vi "Unique.vi"(11 "Type in":refnum<class "Type.lvclass">) -> (2 "Unique":bool)   [LabVIEW 2020, in "Conditum.lvlib" / "Columns.lvlib" / "Type.lvclass"]
uses:
  Type.lvclass
  Type.lvclass/Type.ctl
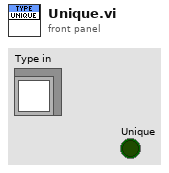
[diagram p1: front panel]
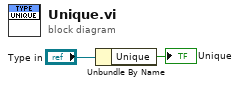
[diagram p0: block diagram]
diagram:
  n1 = Unbundle By Name("Type in") -> ("Unique"=→"Unique":bool)
